vi "RSZVB Get Pulse Generator Polarity.vi"(8 "error in (no error)":errorcluster {"code" format="%.0x"}, 9 "Generator (1)":i32=1, 10 "Channel (1)":i32=1, 11 "VISA session":refnum<visa-resource-name>) -> (0 "error out":errorcluster {"code" format="%.0x"}, 1 "Pulse Polarity":i32, 3 "dup VISA session":refnum<visa-resource-name>)   [LabVIEW 2011]
doc: "This VI returns the polarity of the pulse generator signal <gen_no>. \n\nNote(s):\n\n(1) This VI is available only with option R&S ZVA-K27.\n\nRemote-control command(s):\n[SENSe<Ch>:]PULSe:GENerator<gen_no>:POLarity?"
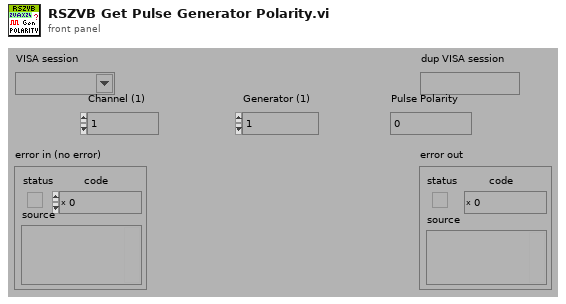
[diagram p1: front panel]
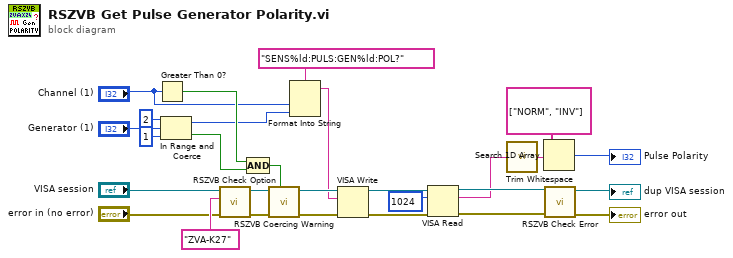
[diagram p0: block diagram]
diagram:
  n1 = Greater Than 0?(x="Channel (1)") -> (x > 0?=w17:bool)
  n2 = In Range and Coerce(upper limit=2, x="Generator (1)", lower limit=1) -> (coerced(x)=w16:i32, In Range?=w18:bool)
  n3 = call "RSZVB Check Option.vi"("error in (no error)"="error in (no error)", "Options"="ZVA-K27", "VISA session"="VISA session") -> ("error out"=w24:errorcluster, "dup VISA session"=w23:refnum<visa-resource-name>)  [unwired: 7 in]
  n4 = Compound Arithmetic op=AND(w17, w18) -> (w20:bool)
  n5 = call "RSZVB Coercing Warning.vi"("In Range?"=w20, "error in (no error)"=w24, "VISA session"=w23) -> ("error out"=w27:errorcluster, "dup VISA session"=w28:refnum<visa-resource-name>)  [unwired: 7 in]
  n6 = Format Into String(format string="SENS%ld:PULS:GEN%ld:POL?", "Channel (1)", w16) -> (resulting string=w26:string)  [unwired: 2 in, 1 out]
  n7 = VISA Write(VISA resource name=w28, write buffer=w26, error in (no error)=w27) -> (VISA resource name out=w14:refnum<visa-resource-name>, error out=w13:errorcluster)  [unwired: 1 out]
  n8 = VISA Read(VISA resource name=w14, byte count=u32 1024 ("byte count (0)"), error in (no error)=w13) -> (VISA resource name out=w12:refnum<visa-resource-name>, read buffer=w9:string, error out=w11:errorcluster)  [unwired: 1 out]
  n9 = call <vilib>:"Trim Whitespace.vi"("string"=w9) -> ("trimmed string"=w8:string)  [unwired: 1 in]
  n10 = Search 1D Array(1D array=string[] ["NORM", "INV"], element=w8) -> (index of element=→"Pulse Polarity":i32)  [unwired: 1 in]
  n11 = call "RSZVB Check Error.vi"("error in (no error)"=w11, "VISA session"=w12) -> ("error out"=→"error out":errorcluster, "dup VISA session"=→"dup VISA session":refnum<visa-resource-name>)  [unwired: 8 in]
